vi "RoomsFGV.vi"(7 "Actions":T1, 8 "error in (no error)":errorcluster, 9 "Data In":string, 10 "Room":i32) -> (0 "error out":errorcluster, 1 "Data Out":string)   [LabVIEW 2015]
uses:
  TypeDef/RoomsActionEnum.ctl
  TypeDef/StateCluster.ctl
  LVClasses/Room/Room.lvclass
  LVClasses/Room/Room.lvclass/Room.ctl
  LVClasses/Flags/Flags.lvclass/Flags.ctl
  LVClasses/Room/Write Bed URL.vi
  LVClasses/Room/Read Flags.lvclass.vi
  LVClasses/Room/Read BedVacant.vi
  LVClasses/Flags/Read State.vi
  LVClasses/Flags/Write State.vi
  LVClasses/Room/Write Flags.lvclass.vi
  LVClasses/Room/Write BedVacant.vi
  LVClasses/Flags/Flags.lvclass
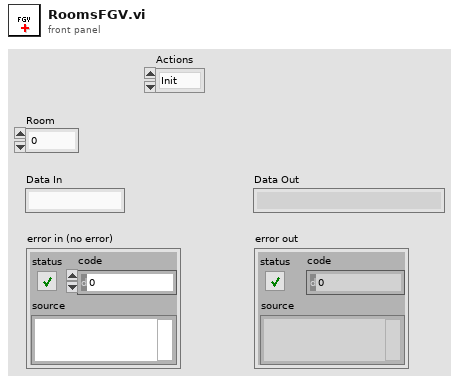
[diagram p1: front panel]
types:
  T1 = typedef "RoomsActionEnum.ctl" = enum16{"Init", "Add Room", "Remove Room", "Read Room", "Read Flag", "Read Flag State", "Write Flag State", "Read Flag Color", "Write Flag Color", "Read Bed Vacant", "Write Bed Vacant", "Read Personnel", "Add Personnel", "Remove Personnel", "Read Requests", "Add Request", "Remove Request", "Read Beacon ID", "Write Beacon ID", "Write Bed URL", "Read Bed URL", "Get Rooms Numbers"}
  T2 = typedef "StateCluster.ctl" = cluster{"Rooms":refnum<class "Room.lvclass">[]}
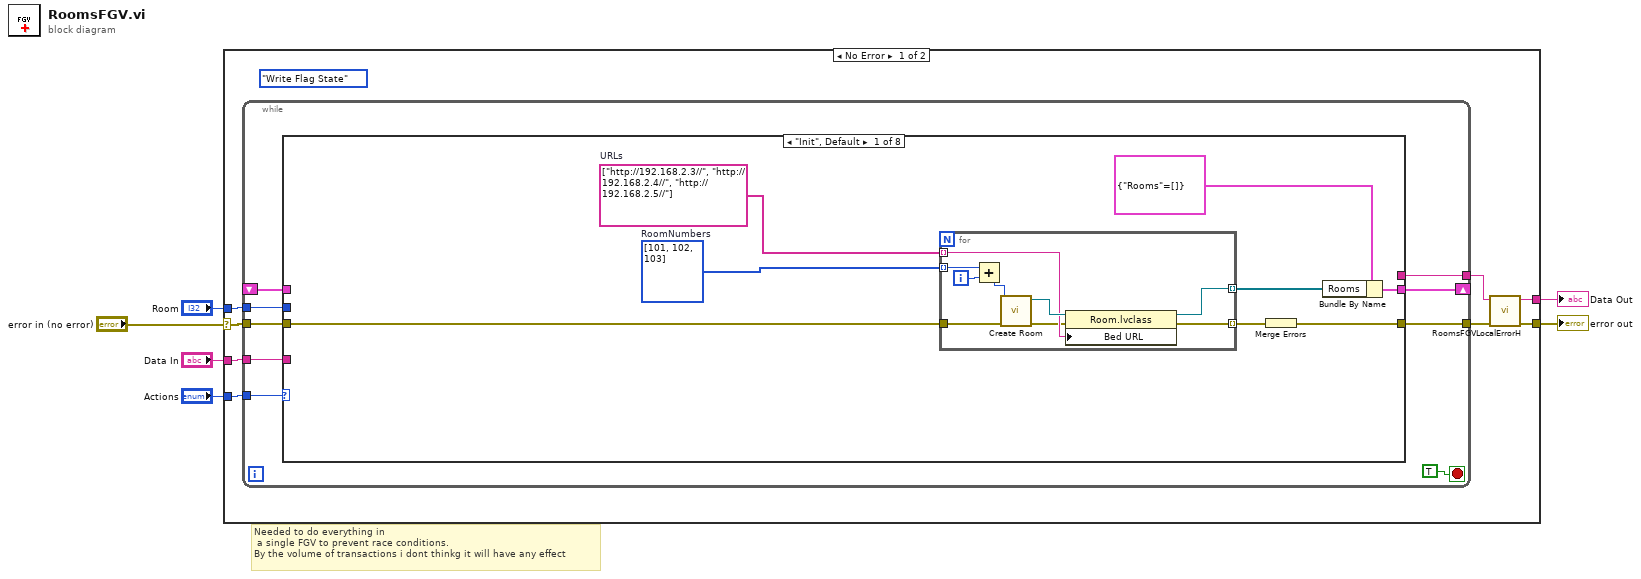
[diagram p0: block diagram]
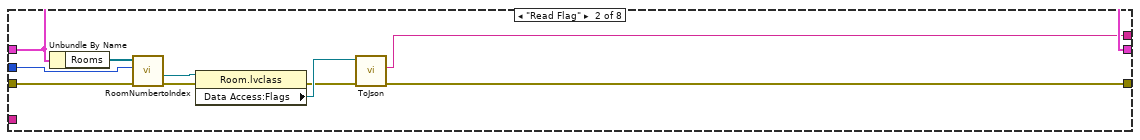
[diagram p2: hidden frame]
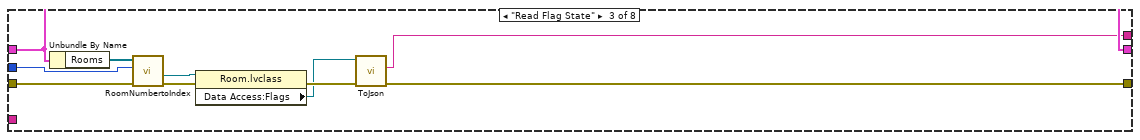
[diagram p3: hidden frame]
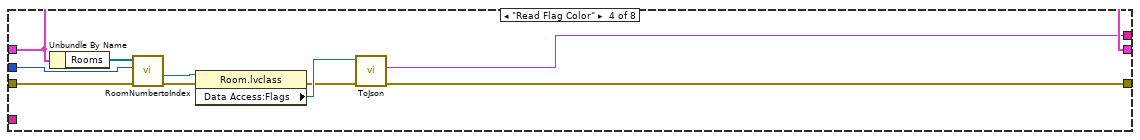
[diagram p4: hidden frame]
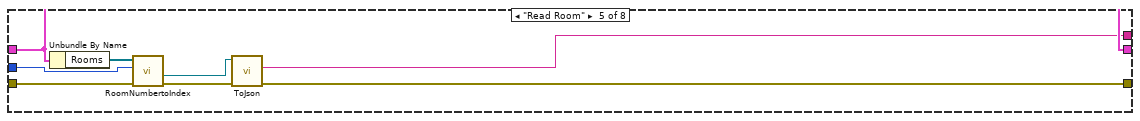
[diagram p5: hidden frame]
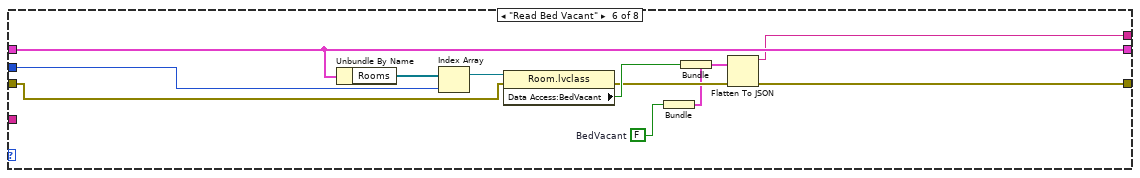
[diagram p6: hidden frame]
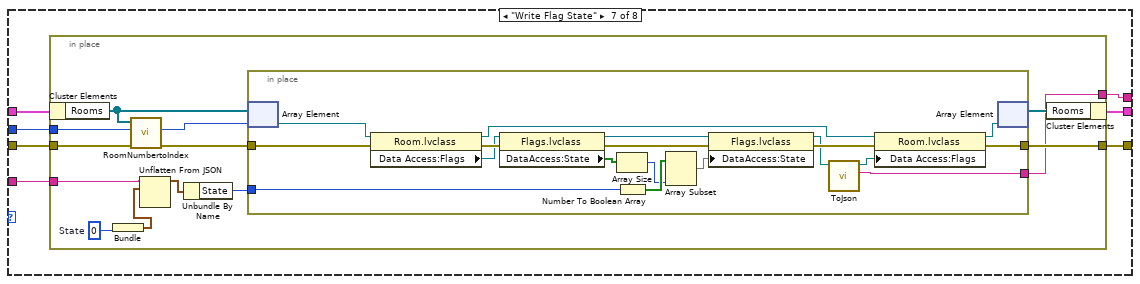
[diagram p7: hidden frame]
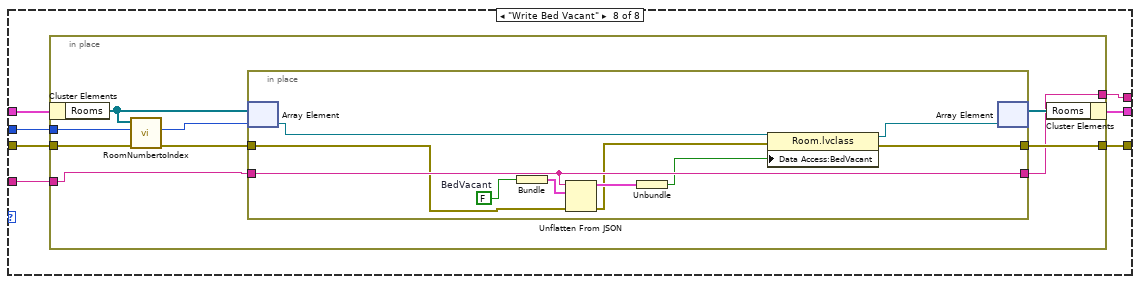
[diagram p8: hidden frame]
diagram:
  # "Needed to do everything in\n a single FGV to prevent race conditions. \nBy the volume of transactions i dont thinkg it will have any effect"
  n1 = case shown="No Error" "error in (no error)" {
    selector: "error in (no error)" -> [w11 w155]
    tunnel: "Actions" -> [w14 _]
    tunnel: "Room" -> [w13 _]
    tunnel: [w8 _] -> w4
    tunnel: "Data In" -> [w12 _]
    tunnel: [w9 w155] -> w1
    frame No Error {
      (unwired) RoomsActionEnum."Write Flag State" ("Actions")
      n2 = while {
        shift-right: [w21] -> _
        shift-left: _ -> [w20]
        tunnel: w14 -> [w22]
        tunnel: w13 -> [w19]
        tunnel: [w18] -> w7
        tunnel: w12 -> [w17]
        tunnel: [w16] -> w10
        tunnel: w11 -> [w15]
        stop <- TRUE ("stop") stop-if-true
        n3 = case shown="\"Init\", Default" w22 {
          tunnel: [w31 w50 w60 w70 w78 w90 w96 w134] -> w21
          tunnel: w20 -> [_ w50 w60 w70 w78 w90 w97 w135]
          tunnel: w19 -> [_ w49 w59 w69 w77 w88 w95 w133]
          tunnel: [_ w44 w54 w64 w72 w85 w94 w132] -> w18
          tunnel: w17 -> [_ _ _ _ _ _ w91 w129]
          tunnel: [w24 w46 w56 w66 w71 w82 w92 w130] -> w16
          tunnel: w15 -> [w25 w45 w55 w65 w75 w81 w93 w131]
          frame "Init", Default {
            w28 = i32[] [101, 102, 103]  # RoomNumbers
            w27 = string[] ["http://192.168.2.3//", "http://192.168.2.4//", "http://192.168.2.5//"]  # URLs
            n4 = for {
              tunnel: w28 -> [w38] mode=indexing
              tunnel: [w36] -> w29 mode=indexing
              tunnel: w27 -> [w35] mode=indexing
              tunnel: w25 -> [w33]
              tunnel: [w32] -> w26 mode=indexing
              i -> [w39]
              n5 = Add(x=w38, y=w39) -> (x+y=w40:i32)
              n6 = call "Create Room.vi"("error in"=w33, "Room Number"=w40) -> ("error out"=w34:errorcluster, "Room Ref"=w37:refnum<class "Room.lvclass">)  [unwired: 8 in]
              n7 = property class="Room.lvclass"(reference=w37, error in=w34, "Bed URL"=w35) -> (reference out=w36:refnum<class "Room.lvclass">, error out=w32:errorcluster)
            }
            n8 = Merge Errors(w26) -> (w24:errorcluster)
            n9 = Bundle By Name(cluster=T2 {"Rooms"=[]}, "Rooms"=w29) -> (w31:T2)
          }
          frame "Read Flag" {
            n10 = Unbundle By Name(w50) -> ("Rooms"=w48:refnum<class "Room.lvclass">[])
            n11 = call "RoomNumbertoIndex.vi"("error in (no error)"=w45, "y"=w49, "Rooms In"=w48) -> ("error out"=w41:errorcluster, "Room"=w47:refnum<class "Room.lvclass">)  [unwired: 5 in, 2 out]
            n12 = property class="Room.lvclass"(reference=w47, error in=w41) -> (error out=w42:errorcluster, "Data Access:Flags"=w43:refnum<class "Flags.lvclass">)  [unwired: 1 out]
            n13 = call "ToJson.vi"("error in (no error)"=w42, "Flags in"=w43) -> ("error out"=w46:errorcluster, "String"=w44:string)  [unwired: 7 in, 1 out]
          }
          frame "Read Flag State" {
            n14 = Unbundle By Name(w60) -> ("Rooms"=w58:refnum<class "Room.lvclass">[])
            n15 = call "RoomNumbertoIndex.vi"("error in (no error)"=w55, "y"=w59, "Rooms In"=w58) -> ("error out"=w52:errorcluster, "Room"=w57:refnum<class "Room.lvclass">)  [unwired: 5 in, 2 out]
            n16 = property class="Room.lvclass"(reference=w57, error in=w52) -> (error out=w53:errorcluster, "Data Access:Flags"=w51:refnum<class "Flags.lvclass">)  [unwired: 1 out]
            n17 = call "ToJson.vi"("error in (no error)"=w53, "Flags in"=w51) -> ("error out"=w56:errorcluster, "String"=w54:string)  [unwired: 7 in, 1 out]
          }
          frame "Read Flag Color" {
            n18 = Unbundle By Name(w70) -> ("Rooms"=w68:refnum<class "Room.lvclass">[])
            n19 = call "RoomNumbertoIndex.vi"("error in (no error)"=w65, "y"=w69, "Rooms In"=w68) -> ("error out"=w61:errorcluster, "Room"=w67:refnum<class "Room.lvclass">)  [unwired: 5 in, 2 out]
            n20 = property class="Room.lvclass"(reference=w67, error in=w61) -> (error out=w62:errorcluster, "Data Access:Flags"=w63:refnum<class "Flags.lvclass">)  [unwired: 1 out]
            n21 = call "ToJson.vi"("error in (no error)"=w62, "Flags in"=w63) -> ("error out"=w66:errorcluster, "String"=w64:string)  [unwired: 7 in, 1 out]
          }
          frame "Read Room" {
            n22 = Unbundle By Name(w78) -> ("Rooms"=w76:refnum<class "Room.lvclass">[])
            n23 = call "RoomNumbertoIndex.vi"("error in (no error)"=w75, "y"=w77, "Rooms In"=w76) -> ("error out"=w74:errorcluster, "Room"=w73:refnum<class "Room.lvclass">)  [unwired: 5 in, 2 out]
            n24 = call "ToJson.vi"("error in (no error)"=w74, "Room in"=w73) -> ("error out"=w71:errorcluster, "String"=w72:string)  [unwired: 7 in, 1 out]
          }
          frame "Read Bed Vacant" {
            w80 = FALSE  # BedVacant
            n25 = Unbundle By Name(w90) -> ("Rooms"=w89:refnum<class "Room.lvclass">[])
            n26 = Index Array(array=w89, index=w88) -> (element=w87:refnum<class "Room.lvclass">)
            n27 = property class="Room.lvclass"(reference=w87, error in=w81) -> (error out=w83:errorcluster, "Data Access:BedVacant"=w84:bool)  [unwired: 1 out]
            n28 = Bundle("BedVacant"=w80) -> (w79:cluster{"BedVacant":bool})  [unwired: 1 in]
            n29 = Bundle(cluster=w79, "BedVacant"=w84) -> (w86:cluster{"BedVacant":bool})
            n30 = Flatten To JSON(anything=w86, error in (no error)=w83) -> (JSON string=w85:string, 11:w82:errorcluster)  [unwired: 1 in]
          }
          frame "Write Flag State" {
            n31 = in-place {
              in-place-border: w95 -> [w108]
              in-place-border: [w104] -> w94
              in-place-border: w93 -> [w106]
              in-place-border: [w105] -> w92
              in-place-border: w91 -> [w102]
              w101 = 0  # State
              n32 = in-place-cluster #1(w97) -> ("Rooms"=w109:refnum<class "Room.lvclass">[])
              n33 = Bundle("State"=w101) -> (w100:cluster{"State":i32})  [unwired: 1 in]
              n34 = call "RoomNumbertoIndex.vi"("error in (no error)"=w106, "y"=w108, "Rooms In"=w109) -> ("error out"=w103:errorcluster, "Index"=w107:i32)  [unwired: 5 in, 2 out]
              n35 = Unflatten From JSON(JSON string=w102, type and defaults=w100) -> (value=w99:cluster{"State":i32})  [unwired: 5 in, 1 out]
              n36 = Unbundle By Name(w99) -> ("State"=w98:i32)
              n37 = in-place {
                in-place-border: w103 -> [w123]
                in-place-border: [w115] -> w105
                in-place-border: w98 -> [w126]
                in-place-border: [w111] -> w104
                n38 = in-place-array #2(w109, w107) -> (w118:refnum<class "Room.lvclass">)
                n39 = property class="Room.lvclass"(reference=w118, error in=w123) -> (reference out=w117:refnum<class "Room.lvclass">, error out=w124:errorcluster, "Data Access:Flags"=w122:refnum<class "Flags.lvclass">)
                n40 = property class="Flags.lvclass"(reference=w122, error in=w124) -> (reference out=w114:refnum<class "Flags.lvclass">, error out=w125:errorcluster, "DataAccess:State"=w121:bool[])
                n41 = Array Size(array=w121) -> (size(s)=w120:i32)
                n42 = Number To Boolean Array(number=w126) -> (Boolean array=w127:bool[])
                n43 = Array Subset(array=w127, length=w120) -> (w119:bool[])  [unwired: 1 in]
                n44 = property class="Flags.lvclass"(reference=w114, error in=w125, "DataAccess:State"=w119) -> (reference out=w113:refnum<class "Flags.lvclass">, error out=w116:errorcluster)
                n45 = call "ToJson.vi"("Flags in"=w113) -> ("String"=w111:string, "Flags out"=w112:refnum<class "Flags.lvclass">)  [unwired: 8 in, 1 out]
                n46 = property class="Room.lvclass"(reference=w117, error in=w116, "Data Access:Flags"=w112) -> (reference out=w128:refnum<class "Room.lvclass">, error out=w115:errorcluster)
                n47 = in-place-array #2(w128) -> (w110:refnum<class "Room.lvclass">[])  [unwired: 1 out]
              }
              n48 = in-place-cluster #1("Rooms"=w110) -> (w96:T2)
            }
          }
          frame "Write Bed Vacant" {
            n49 = in-place {
              in-place-border: w133 -> [w142]
              in-place-border: [w138] -> w132
              in-place-border: w131 -> [w140]
              in-place-border: [w139] -> w130
              in-place-border: w129 -> [w137]
              n50 = in-place-cluster #3(w135) -> ("Rooms"=w143:refnum<class "Room.lvclass">[])
              n51 = call "RoomNumbertoIndex.vi"("error in (no error)"=w140, "y"=w142, "Rooms In"=w143) -> ("error out"=w136:errorcluster, "Index"=w141:i32)  [unwired: 5 in, 2 out]
              n52 = in-place {
                in-place-border: w136 -> [w145]
                in-place-border: [w154] -> w139
                in-place-border: [w151] -> w138
                in-place-border: w137 -> [w151]
                w148 = FALSE  # BedVacant
                n53 = in-place-array #4(w143, w141) -> (w147:refnum<class "Room.lvclass">)
                n54 = Bundle("BedVacant"=w148) -> (w152:cluster{"BedVacant":bool})  [unwired: 1 in]
                n55 = Unflatten From JSON(JSON string=w151, type and defaults=w152, error in (no error)=w145) -> (value=w150:cluster{"BedVacant":bool}, error out=w146:errorcluster)  [unwired: 4 in]
                n56 = Unbundle(w150) -> ("BedVacant"=w149:bool)
                n57 = property class="Room.lvclass"(reference=w147, error in=w146, "Data Access:BedVacant"=w149) -> (reference out=w153:refnum<class "Room.lvclass">, error out=w154:errorcluster)
                n58 = in-place-array #4(w153) -> (w144:refnum<class "Room.lvclass">[])  [unwired: 1 out]
              }
              n59 = in-place-cluster #3("Rooms"=w144) -> (w134:T2)
            }
          }
        }
      }
      n60 = call "RoomsFGVLocalErrorH.vi"("error in (no error)"=w10, "String in"=w7) -> ("error out"=w9:errorcluster, "String out"=w8:string)  [unwired: 8 in]
    }
    frame Error {
    }
  }
  "Data Out" <- w4
  "error out" <- w1
